vi "AWG Set and Arm.vi"(7 "pulse count (0: infinite)":i32, 8 "error in (no error)":errorcluster, 9 "trigger":T1, 10 "sampling rate":T5={"freq mode"=enum."fs or Ts", "fs [Hz]"=0.0, "fref [Hz]"=0.0, "mul"=0.0, "div"=0.0, "Amplitude (V)"=1.0}, 11 "awg session in":T7={"type"=enum."Agilent 331xxA to 332xxA", "VISA"="", "enable 10MHz ref"=FALSE, "cmi ckd2"={"VISA"="", "clock source"=enum."Auto", "manual ref clk"=FALSE, "ref clock [Hz]"=0.0, "div mode"=enum."Set divisor directly"}, "cmi sync v3"={"VISA"="", "baud rate [bd/s]"=115200, "source"=enum."Auto", "hv range"=enum."1kV", "fsrc is fixed"=FALSE, "fsrc [Hz]"=10000000.0, "freq integ [s]"=1.0, "freq filter"=5, "trig level"=enum."TTL 5V", "chn1 mode"=enum."Source divider", "chn1 level"=enum."Positive 5V", "chn2 mode"=enum."Source divider", "chn2 level"=enum."Positive 5V", "chn2 div"=1, "chn3 mode"=enum."Chn 1 Active", "chn3 level"=enum."Positive 5V", "chn1 div entry"=enum."Calculate nearest divisor from measured fx", "chn1 dev limit [%]"=1.0, "chn1 check dev"=FALSE}, "trigger"={"source"=enum."Immediate", "level [V]"=0.0, "coupling"=enum."DC", "slope"=enum."POS"}, "HMF2500 cfg"={"Baud Rate"=9600, "Parity"=0, "Data Bits"=8, "Flow Control"=4}} {"HMF2500 cfg"."Flow Control" items=["None", "XON/XOFF", "RTS/CTS", "XON/XOFF & RTS/CTS", "DTR/DSR", "XON/XOFF & DTR/DSR"]; "HMF2500 cfg"."Data Bits" items=["7"=7, "8"=8]; "HMF2500 cfg"."Parity" items=["None", "Odd", "Even", "Mark", "Space"]; "HMF2500 cfg"."Baud Rate" items=["300"=300, "600"=600, "1200"=1200, "2400"=2400, "4800"=4800, "9600"=9600, "19200"=19200]; "cmi sync v3"."chn2 div" min=1 max=100000000 step=1; "cmi sync v3"."fsrc [Hz]" format="%_8p"}) -> (0 "error out":errorcluster, 3 "awg session out":T7={"type"=enum."Agilent 331xxA to 332xxA", "VISA"="", "enable 10MHz ref"=FALSE, "cmi ckd2"={"VISA"="", "clock source"=enum."Auto", "manual ref clk"=FALSE, "ref clock [Hz]"=0.0, "div mode"=enum."Set divisor directly"}, "cmi sync v3"={"VISA"="", "baud rate [bd/s]"=115200, "source"=enum."Auto", "hv range"=enum."1kV", "fsrc is fixed"=FALSE, "fsrc [Hz]"=10000000.0, "freq integ [s]"=1.0, "freq filter"=5, "trig level"=enum."TTL 5V", "chn1 mode"=enum."Source divider", "chn1 level"=enum."Positive 5V", "chn2 mode"=enum."Source divider", "chn2 level"=enum."Positive 5V", "chn2 div"=1, "chn3 mode"=enum."Chn 1 Active", "chn3 level"=enum."Positive 5V", "chn1 div entry"=enum."Calculate nearest divisor from measured fx", "chn1 dev limit [%]"=1.0, "chn1 check dev"=FALSE}, "trigger"={"source"=enum."Immediate", "level [V]"=0.0, "coupling"=enum."DC", "slope"=enum."POS"}, "HMF2500 cfg"={"Baud Rate"=9600, "Parity"=0, "Data Bits"=8, "Flow Control"=4}} {"HMF2500 cfg"."Flow Control" items=["None", "XON/XOFF", "RTS/CTS", "XON/XOFF & RTS/CTS", "DTR/DSR", "XON/XOFF & DTR/DSR"]; "HMF2500 cfg"."Data Bits" items=["7"=7, "8"=8]; "HMF2500 cfg"."Parity" items=["None", "Odd", "Even", "Mark", "Space"]; "HMF2500 cfg"."Baud Rate" items=["300"=300, "600"=600, "1200"=1200, "2400"=2400, "4800"=4800, "9600"=9600, "19200"=19200]; "cmi sync v3"."chn2 div" min=1 max=100000000 step=1; "cmi sync v3"."fsrc [Hz]" format="%_8p"})   [LabVIEW 2020, in "AWG.lvlib"]
doc: "AWG wrapper: This sets the AWG to desired frequency and arms it. No pulses are generated here. Waiting for trigger!"
uses:
  AWG.lvlib
  AWG Session.ctl
  AWG Type.ctl
  CMI Clock Divider v2/CMI ckd2 Session.ctl
  CMI Clock Divider v2/CMI ckd2 Source Mode.ctl
  CMI Clock Divider v2/CMI ckd2 Divisor Mode.ctl
  CMI Sync V3/CMI Sync V3 session.ctl
  CMI Sync V3/Configure/CMI Sync V3 Reference Clock Source.ctl
  CMI Sync V3/Configure/CMI Sync V3 HV input Range.ctl
  CMI Sync V3/Configure/CMI Sync V3 Trigger Input Level.ctl
  CMI Sync V3/Configure/CMI Sync V3 Channel 1 Mode.ctl
  CMI Sync V3/Configure/CMI Sync V3 Channel Output Levels.ctl
  CMI Sync V3/Configure/CMI Sync V3 Channel 2 Mode.ctl
  CMI Sync V3/Configure/CMI Sync V3 Channel 3 Mode.ctl
  CMI Sync V3/Configure/CMI Sync V3 Channel 1 Divisor Entry Mode.ctl
  externals needed for AWG/ADC Trig Config.ctl
  externals needed for AWG/ADC Trig Mode Source.ctl
  externals needed for AWG/ADC Trig Coupling.ctl
  externals needed for AWG/ADC Trig Slope.ctl
  RaS HMF2500/HMF2500 Config.ctl
  externals needed for AWG/3458A Sampling Rate.ctl
  AWG Clock Setup Mode.ctl
  Agilent 33XXX Series/Agilent 33XXX Series.lvlib
  AFG3000/Tektronix AFG 3000 Series.lvlib
  CMI Sync V3/CMI Sync Unit V3.lvlib
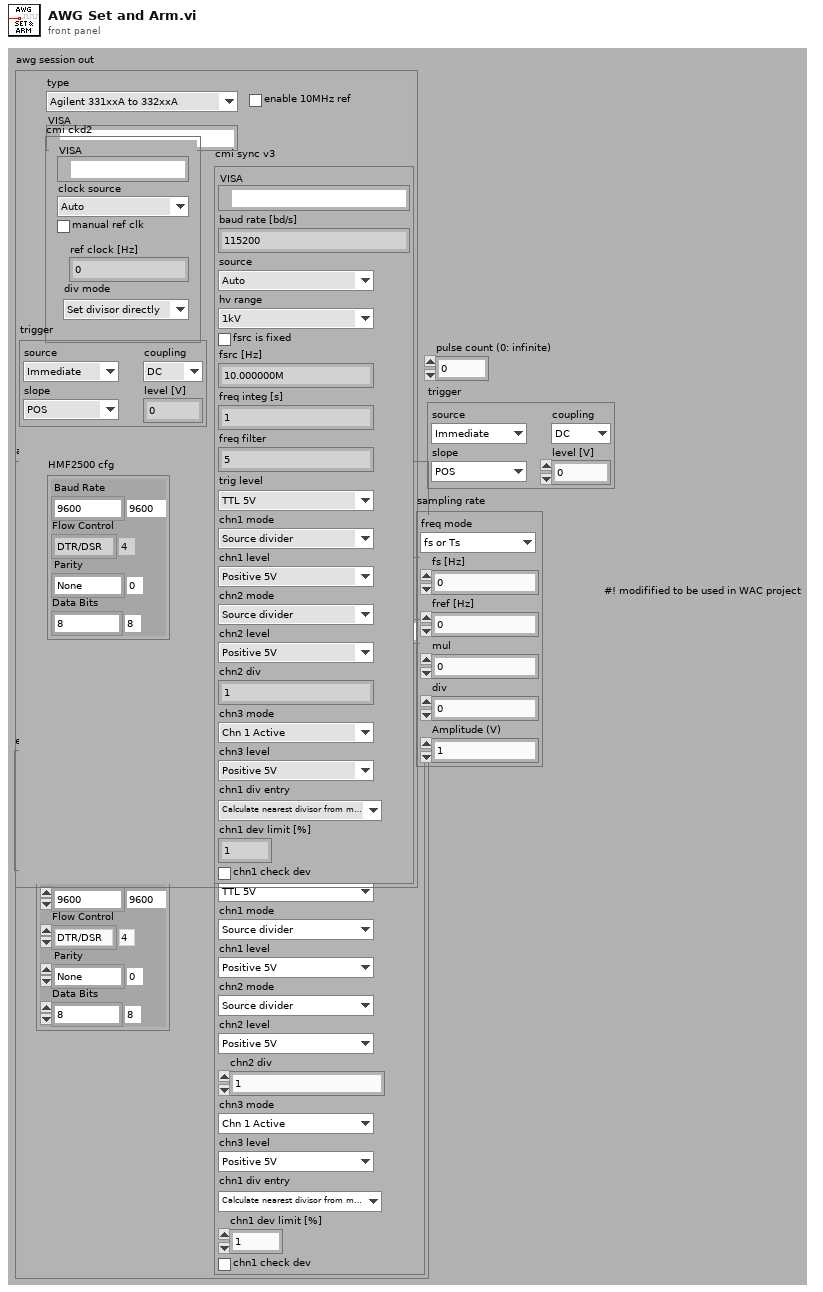
[diagram p1: front panel]
types:
  T1 = typedef "ADC Trig Config.ctl" = cluster{"source":T2, "level [V]":dbl, "coupling":T3, "slope":T4}
  T2 = typedef "ADC Trig Mode Source.ctl" = enum16{"Immediate", "External", "Level"}
  T3 = typedef "ADC Trig Coupling.ctl" = enum16{"DC", "AC"}
  T4 = typedef "ADC Trig Slope.ctl" = enum16{"POS", "NEG"}
  T5 = typedef "3458A Sampling Rate.ctl" = cluster{"freq mode":T6, "fs [Hz]":dbl, "fref [Hz]":dbl, "mul":dbl, "div":dbl, "Amplitude (V)":dbl}
  T6 = typedef "AWG.lvlib/AWG Clock Setup Mode.ctl" = enum16{"fs or Ts", "fs or Ts with fref", "fref/N", "fref*M/N", "fref*Ratio"}
  T7 = typedef "AWG.lvlib/AWG Session.ctl" = cluster{"type":T8, "VISA":refnum<visa-resource-name>, "enable 10MHz ref":bool, "cmi ckd2":T9, "cmi sync v3":T12, "trigger":T1, "HMF2500 cfg":T21}
  T8 = typedef "AWG.lvlib/AWG Type.ctl" = enum16{"Agilent 331xxA to 332xxA", "Agilent 335xxA to 336xxA", "Tektronix AFG3101C", "R&S HMF25xx", "CMI Clock Divider v2", "CMI Sync Unit V3", "dummy"}
  T9 = typedef "AWG.lvlib/CMI ckd2 Session.ctl" = cluster{"VISA":refnum<visa-resource-name>, "clock source":T10, "manual ref clk":bool, "ref clock [Hz]":dbl, "div mode":T11}
  T10 = typedef "AWG.lvlib/CMI ckd2 Source Mode.ctl" = enum16{"Auto", "LF clock", "HF clock", "Internal"}
  T11 = typedef "AWG.lvlib/CMI ckd2 Divisor Mode.ctl" = enum16{"Set divisor directly", "Set divisor by frequency"}
  T12 = typedef "AWG.lvlib/CMI Sync Unit V3.lvlib/CMI Sync V3 session.ctl" = cluster{"VISA":refnum<visa-resource-name>, "baud rate [bd/s]":i32, "source":T13, "hv range":T14, "fsrc is fixed":bool, "fsrc [Hz]":dbl, "freq integ [s]":dbl, "freq filter":i32, "trig level":T15, "chn1 mode":T16, "chn1 level":T17, "chn2 mode":T18, "chn2 level":T17, "chn2 div":i32, "chn3 mode":T19, "chn3 level":T17, "chn1 div entry":T20, "chn1 dev limit [%]":dbl, "chn1 check dev":bool}
  T13 = typedef "AWG.lvlib/CMI Sync Unit V3.lvlib/CMI Sync V3 Reference Clock Source.ctl" = enum16{"Auto", "Internal", "Logic", "Sine", "HV"}
  T14 = typedef "AWG.lvlib/CMI Sync Unit V3.lvlib/CMI Sync V3 HV input Range.ctl" = enum16{"10V", "60V", "250V", "1kV"}
  T15 = typedef "AWG.lvlib/CMI Sync Unit V3.lvlib/CMI Sync V3 Trigger Input Level.ctl" = enum16{"LVCMOS 3V3", "TTL 5V"}
  T16 = typedef "AWG.lvlib/CMI Sync Unit V3.lvlib/CMI Sync V3 Channel 1 Mode.ctl" = enum16{"Source divider", "DDS absolute", "DDS ratio", "DDS ratio M/N"}
  T17 = typedef "AWG.lvlib/CMI Sync Unit V3.lvlib/CMI Sync V3 Channel Output Levels.ctl" = enum16{"Positive 3V3", "Negative 3V3", "Positive 5V", "Negative 5V"}
  T18 = typedef "AWG.lvlib/CMI Sync Unit V3.lvlib/CMI Sync V3 Channel 2 Mode.ctl" = enum16{"Source divider", "Chn 1 divide"}
  T19 = typedef "AWG.lvlib/CMI Sync Unit V3.lvlib/CMI Sync V3 Channel 3 Mode.ctl" = enum16{"Chn 1 Active", "Chn 2 Active", "Chn 1 Trigger", "Chn 2 Trigger", "Gate", "PPS", "10MHz"}
  T20 = typedef "AWG.lvlib/CMI Sync Unit V3.lvlib/CMI Sync V3 Channel 1 Divisor Entry Mode.ctl" = enum16{"Set divisor directly", "Calculate nearest divisor from measured fx"}
  T21 = typedef "AWG.lvlib/HMF2500 Config.ctl" = cluster{"Baud Rate":u32, "Parity":u16, "Data Bits":u16, "Flow Control":u16}
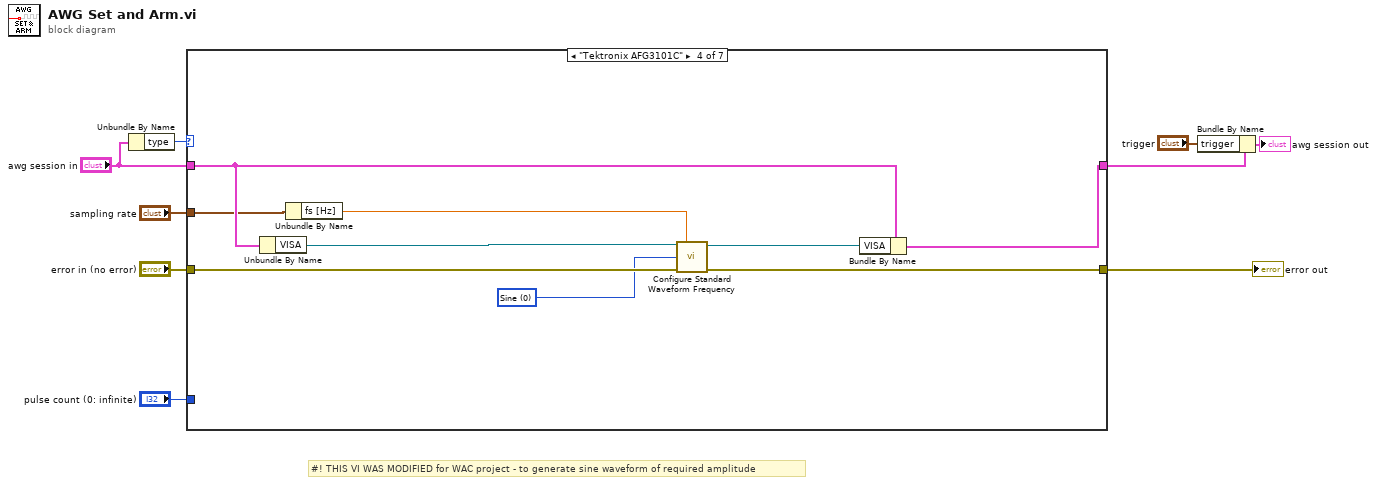
[diagram p0: block diagram]
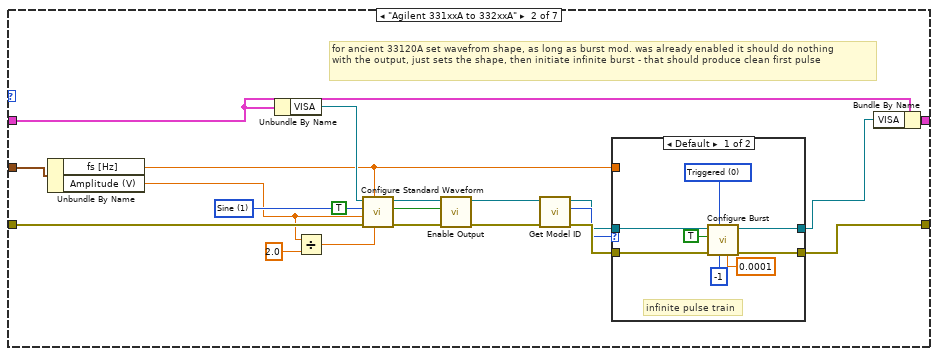
[diagram p3: hidden frame]
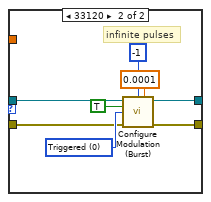
[diagram p4: hidden frame]
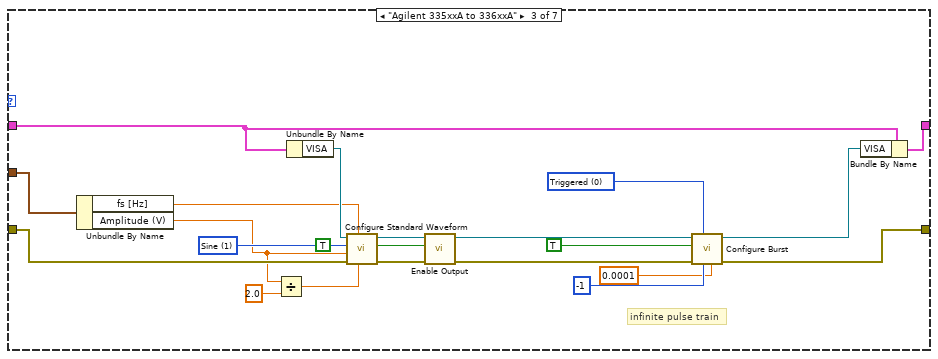
[diagram p5: hidden frame]
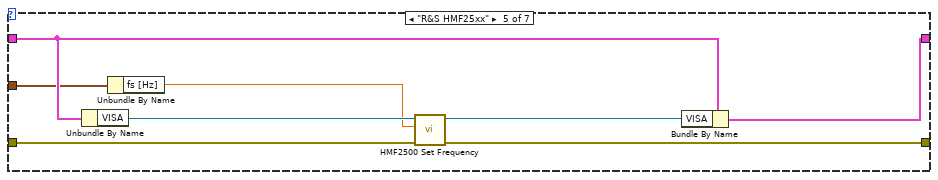
[diagram p6: hidden frame]
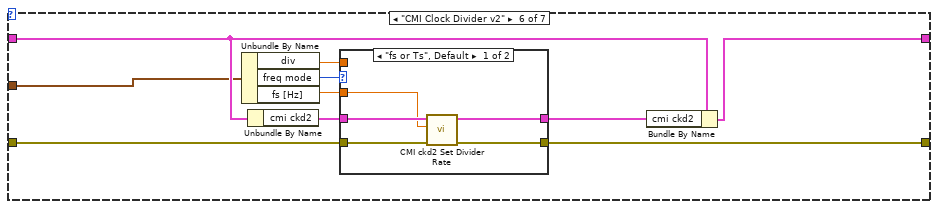
[diagram p7: hidden frame]
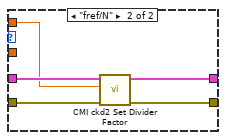
[diagram p8: hidden frame]
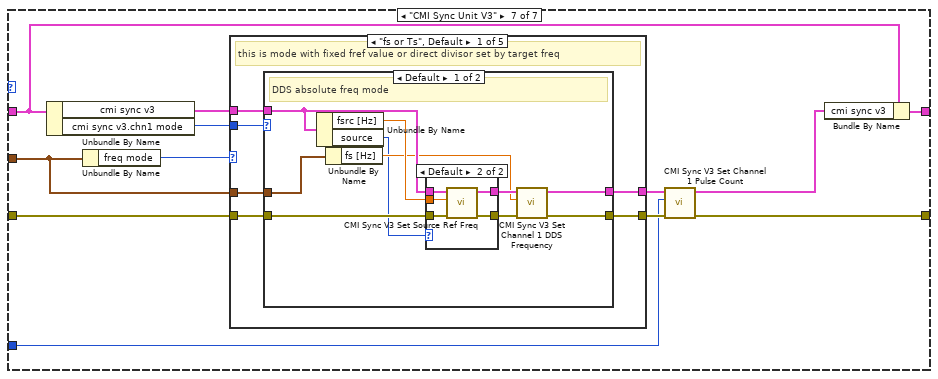
[diagram p9: hidden frame]
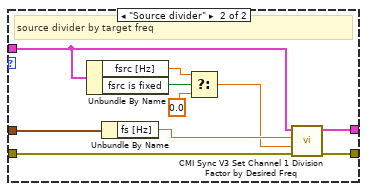
[diagram p11: hidden frame]
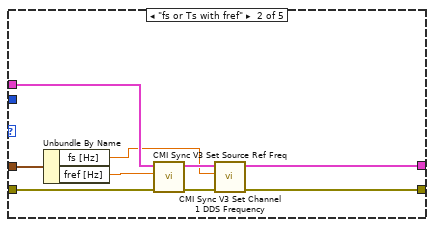
[diagram p12: hidden frame]
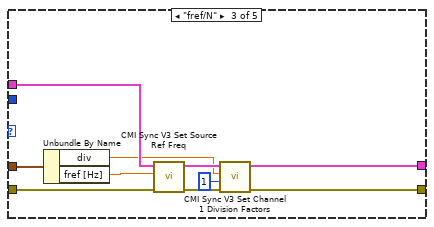
[diagram p13: hidden frame]
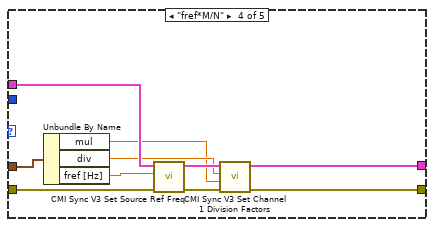
[diagram p14: hidden frame]
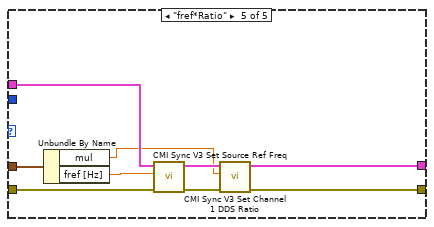
[diagram p15: hidden frame]
diagram:
  # "#! THIS VI WAS MODIFIED for WAC project - to generate sine waveform of required amplitude"
  n1 = Unbundle By Name("awg session in") -> ("type"=w9:T8)
  n2 = case shown="\"Tektronix AFG3101C\"" w9 {
    tunnel: "error in (no error)" -> [w11 w27 w60 w74 w82 w95 w116]
    tunnel: [w11 w17 w53 w71 w80 w90 w110] -> w7
    tunnel: "awg session in" -> [w10 w30 w68 w77 w85 w93 w112]
    tunnel: [w10 w31 w67 w76 w84 w89 w113] -> w4
    tunnel: "sampling rate" -> [_ w18 w61 w70 w79 w91 w114]
    tunnel: "pulse count (0: infinite)" -> [_ _ _ _ _ _ w109]
    frame Default {
    }
    frame "Agilent 331xxA to 332xxA" {
      w29 = u16 1 items=["DC", "Sine", "Square", "Triangle", "Ramp", "Pulse", "Noise", "Sinc", "Negative Ramp", "Exponential Rise", "Exponential Fall", "Cardiac"] ("Waveform Function (1: Sine)")
      # "for ancient 33120A set wavefrom shape, as long as burst mod. was already enabled it should do nothing\nwith the output, just sets the shape, then initiate infinite burst - that should produce clean first pulse"
      n3 = Unbundle By Name(w18) -> ("fs [Hz]"=w15:dbl, "Amplitude (V)"=w13:dbl)
      n4 = Unbundle By Name(w30) -> ("VISA"=w28:refnum<visa-resource-name>)
      n5 = Divide(x=w13, y=2.0 ("DC Offset (0.00 V)")) -> (x/y=w12:dbl)
      n6 = call "Configure Standard Waveform.vi"("DC Offset (0.00 V)"=w12, "Frequency (1000 Hz)"=w15, "error in (no error)"=w27, "Amplitude (1)"=w13, "Waveform Function (1: Sine)"=w29, "VISA resource name"=w28) -> ("error out"=w26:errorcluster, "VISA resource name out"=w25:refnum<visa-resource-name>)  [unwired: 4 in]
      n7 = call "Enable Output.vi"("error in (no error)"=w26, "Enable Output  (T: Enable)"=TRUE, "VISA resource name"=w25) -> ("error out"=w23:errorcluster, "VISA resource name out"=w22:refnum<visa-resource-name>)  [unwired: 7 in]
      n8 = call "Get Model ID.vi"("error in (no error)"=w23, "VISA resource name"=w22) -> ("error out"=w21:errorcluster, "model ID"=w20:u32, "VISA resource name out"=w19:refnum<visa-resource-name>)  [unwired: 7 in]
      n9 = case shown="Default" w20 {
        tunnel: [w38 w44] -> w17
        tunnel: [w37 w43] -> w16
        tunnel: w15 -> [_ _]
        tunnel: w21 -> [w39 w42]
        tunnel: w19 -> [w36 w41]
        frame Default {
          w35 = u16 0 items=["Triggered", "Gated"] ("Burst Mode (0: Triggered)")
          # "infinite pulse train"
          n10 = call "Configure Burst.vi"("Burst Period (1 s)"=0.0001, "Burst Count (1)"=-1, "Burst Mode (0: Triggered)"=w35, "error in (no error)"=w39, "Enable Burst (T: Enable)"=TRUE, "VISA resource name"=w36) -> ("error out"=w38:errorcluster, "VISA resource name out"=w37:refnum<visa-resource-name>)  [unwired: 4 in]
        }
        frame 33120 {
          w45 = u16 0 items=["Triggered", "Gated"] ("Burst Modulation Mode (0: Triggered)")
          # "infinite pulses"
          n11 = call "Configure Modulation (Burst).vi"("VISA resource name"=w41, "Burst Count (1)"=-1, "Burst Period (1 s)"=0.0001, "Enable Burst Modulation (T: Enable)"=TRUE, "Burst Modulation Mode (0: Triggered)"=w45, "error in (no error)"=w42) -> ("VISA resource name out"=w43:refnum<visa-resource-name>, "error out"=w44:errorcluster)  [unwired: 8 in]
        }
      }
      n12 = Bundle By Name(cluster=w30, "VISA"=w16) -> (w31:T7)
    }
    frame "Agilent 335xxA to 336xxA" {
      w59 = u16 0 items=["Triggered", "Gated"] ("Burst Mode (0: Triggered)")
      w66 = u16 1 items=["DC", "Sine", "Square", "Triangle", "Ramp", "Pulse", "Noise", "Sinc", "Negative Ramp", "Exponential Rise", "Exponential Fall", "Cardiac"] ("Waveform Function (1: Sine)")
      # "infinite pulse train"
      n13 = Unbundle By Name(w61) -> ("fs [Hz]"=w51:dbl, "Amplitude (V)"=w49:dbl)
      n14 = Divide(x=w49, y=2.0 ("DC Offset (0.00 V)")) -> (x/y=w48:dbl)
      n15 = Unbundle By Name(w68) -> ("VISA"=w62:refnum<visa-resource-name>)
      n16 = call "Configure Standard Waveform.vi"("DC Offset (0.00 V)"=w48, "Frequency (1000 Hz)"=w51, "error in (no error)"=w60, "Amplitude (1)"=w49, "Waveform Function (1: Sine)"=w66, "VISA resource name"=w62) -> ("error out"=w65:errorcluster, "VISA resource name out"=w64:refnum<visa-resource-name>)  [unwired: 4 in]
      n17 = call "Enable Output.vi"("error in (no error)"=w65, "Enable Output  (T: Enable)"=TRUE, "VISA resource name"=w64) -> ("error out"=w55:errorcluster, "VISA resource name out"=w54:refnum<visa-resource-name>)  [unwired: 7 in]
      n18 = call "Configure Burst.vi"("Burst Period (1 s)"=0.0001, "Burst Count (1)"=-1, "Burst Mode (0: Triggered)"=w59, "error in (no error)"=w55, "Enable Burst (T: Enable)"=TRUE, "VISA resource name"=w54) -> ("error out"=w53:errorcluster, "VISA resource name out"=w52:refnum<visa-resource-name>)  [unwired: 4 in]
      n19 = Bundle By Name(cluster=w68, "VISA"=w52) -> (w67:T7)
    }
    frame "Tektronix AFG3101C" {
      w73 = u16 0 items=["Sine", "Square", "Pulse", "Ramp", "Noise", "DC", "Sin(x)/x", "Gaussian", "Lorentz", "Exponential Rise", "Exponential Decay", "Haversine"] ("Waveform Function (0: Sine)")
      n20 = Unbundle By Name(w77) -> ("VISA"=w75:refnum<visa-resource-name>)
      n21 = Unbundle By Name(w70) -> ("fs [Hz]"=w69:dbl)
      n22 = call "Configure Standard Waveform Frequency.vi"("VISA resource name"=w75, "Frequency (1000 Hz)"=w69, "Waveform Function (0: Sine)"=w73, "error in (no error)"=w74) -> ("VISA resource name out"=w72:refnum<visa-resource-name>, "error out"=w71:errorcluster)  [unwired: 10 in]
      n23 = Bundle By Name(cluster=w77, "VISA"=w72) -> (w76:T7)
    }
    frame "R&S HMF25xx" {
      n24 = Unbundle By Name(w85) -> ("VISA"=w83:refnum<visa-resource-name>)
      n25 = Unbundle By Name(w79) -> ("fs [Hz]"=w78:dbl)
      n26 = call "HMF2500 Set Frequency.vi"("error in (no error)"=w82, "frequency [Hz] (1000)"=w78, "VISA in"=w83) -> ("error out"=w80:errorcluster, "VISA out"=w81:refnum<visa-resource-name>)  [unwired: 7 in]
      n27 = Bundle By Name(cluster=w85, "VISA"=w81) -> (w84:T7)
    }
    frame "CMI Clock Divider v2" {
      n28 = Unbundle By Name(w91) -> ("div"=w86:dbl, "freq mode"=w87:T6, "fs [Hz]"=w88:dbl)
      n29 = Unbundle By Name(w93) -> ("cmi ckd2"=w94:T9)
      n30 = case shown="\"fs or Ts\", Default" w87 {
        tunnel: w95 -> [w100 w105]
        tunnel: w94 -> [w98 w102]
        tunnel: [w96 w103] -> w92
        tunnel: [w99 w104] -> w90
        tunnel: w88 -> [w97 _]
        tunnel: w86 -> [_ w101]
        frame "fs or Ts", Default {
          n31 = call "CMI ckd2 Set Divider Rate.vi"("error in"=w100, "clock rate [Hz]"=w97, "session"=w98) -> ("error out"=w99:errorcluster, "session out"=w96:T9)  [unwired: 5 in, 2 out]
        }
        frame "fref/N" {
          n32 = call "CMI ckd2 Set Divider Factor.vi"("error in"=w105, "division factor (1)"=w101, "session"=w102) -> ("error out"=w104:errorcluster, "session out"=w103:T9)  [unwired: 7 in]
        }
      }
      n33 = Bundle By Name(cluster=w93, "cmi ckd2"=w92) -> (w89:T7)
    }
    frame "CMI Sync Unit V3" {
      n34 = Unbundle By Name(w112) -> ("cmi sync v3"=w115:T12, "cmi sync v3.chn1 mode"=w106:T16)
      n35 = Unbundle By Name(w114) -> ("freq mode"=w117:T6)
      n36 = case shown="\"fs or Ts\", Default" w117 {
        tunnel: w116 -> [w123 w159 w169 w179 w188]
        tunnel: w115 -> [w119 w158 w168 w178 w187]
        tunnel: w114 -> [w122 w156 w166 w176 w185]
        tunnel: [w121 w153 w163 w173 w182] -> w111
        tunnel: [w120 w152 w162 w172 w181] -> w108
        tunnel: w106 -> [w118 _ _ _ _]
        frame "fs or Ts", Default {
          # "this is mode with fixed fref value or direct divisor set by target freq"
          n37 = case shown="Default" w118 {
            tunnel: w123 -> [w133 w150]
            tunnel: w122 -> [w131 w149]
            tunnel: [w129 w147] -> w121
            tunnel: [w128 w146] -> w120
            tunnel: w119 -> [w127 w145]
            frame Default {
              # "DDS absolute freq mode"
              n38 = Unbundle By Name(w127) -> ("fsrc [Hz]"=w126:dbl, "source"=w124:T13)
              n39 = Unbundle By Name(w131) -> ("fs [Hz]"=w125:dbl)
              n40 = case shown="Default" w124 {
                tunnel: w133 -> [w135 w140]
                tunnel: [w135 w139] -> w132
                tunnel: [w134 w138] -> w130
                tunnel: w127 -> [w134 w137]
                tunnel: w126 -> [_ w136]
                frame "Internal" {
                }
                frame Default {
                  n41 = call "CMI Sync V3 Set Source Ref Freq.vi"("error in"=w140, "Expected reference frequency [Hz]"=w136, "session in"=w137) -> ("error out"=w139:errorcluster, "session out"=w138:T12)  [unwired: 7 in]
                }
              }
              n42 = call "CMI Sync V3 Set Channel 1 DDS Frequency.vi"("error in"=w132, "DDS absolute [Hz] (1 MHz)"=w125, "session in"=w130) -> ("error out"=w129:errorcluster, "session out"=w128:T12)  [unwired: 7 in]
            }
            frame "Source divider" {
              # "source divider by target freq"
              n43 = Unbundle By Name(w145) -> ("fsrc [Hz]"=w143:dbl, "fsrc is fixed"=w144:bool)
              n44 = Unbundle By Name(w149) -> ("fs [Hz]"=w148:dbl)
              n45 = Select(t=w143, s=w144, f=0.0) -> (s? t:f=w141:dbl)
              n46 = call "CMI Sync V3 Set Channel 1 Division Factor by Desired Freq.vi"("error in"=w150, "explicit ref freq [Hz] (0: auto estimate)"=w141, "target output freq [Hz]"=w148, "session in"=w145) -> ("error out"=w147:errorcluster, "session out"=w146:T12)  [unwired: 4 in, 2 out]
            }
          }
        }
        frame "fs or Ts with fref" {
          n47 = Unbundle By Name(w156) -> ("fs [Hz]"=w151:dbl, "fref [Hz]"=w155:dbl)
          n48 = call "CMI Sync V3 Set Source Ref Freq.vi"("error in"=w159, "Expected reference frequency [Hz]"=w155, "session in"=w158) -> ("error out"=w157:errorcluster, "session out"=w154:T12)  [unwired: 7 in]
          n49 = call "CMI Sync V3 Set Channel 1 DDS Frequency.vi"("error in"=w157, "DDS absolute [Hz] (1 MHz)"=w151, "session in"=w154) -> ("error out"=w153:errorcluster, "session out"=w152:T12)  [unwired: 7 in]
        }
        frame "fref/N" {
          n50 = Unbundle By Name(w166) -> ("div"=w161:dbl, "fref [Hz]"=w165:dbl)
          n51 = call "CMI Sync V3 Set Source Ref Freq.vi"("error in"=w169, "Expected reference frequency [Hz]"=w165, "session in"=w168) -> ("error out"=w167:errorcluster, "session out"=w164:T12)  [unwired: 7 in]
          n52 = call "CMI Sync V3 Set Channel 1 Division Factors.vi"("error in"=w167, "DDS multiplier (1)"=1, "Divider (10)"=w161, "session in"=w164) -> ("error out"=w163:errorcluster, "session out"=w162:T12)  [unwired: 6 in]
        }
        frame "fref*M/N" {
          n53 = Unbundle By Name(w176) -> ("mul"=w170:dbl, "div"=w171:dbl, "fref [Hz]"=w175:dbl)
          n54 = call "CMI Sync V3 Set Source Ref Freq.vi"("error in"=w179, "Expected reference frequency [Hz]"=w175, "session in"=w178) -> ("error out"=w177:errorcluster, "session out"=w174:T12)  [unwired: 7 in]
          n55 = call "CMI Sync V3 Set Channel 1 Division Factors.vi"("error in"=w177, "DDS multiplier (1)"=w170, "Divider (10)"=w171, "session in"=w174) -> ("error out"=w173:errorcluster, "session out"=w172:T12)  [unwired: 6 in]
        }
        frame "fref*Ratio" {
          n56 = Unbundle By Name(w185) -> ("mul"=w180:dbl, "fref [Hz]"=w184:dbl)
          n57 = call "CMI Sync V3 Set Source Ref Freq.vi"("error in"=w188, "Expected reference frequency [Hz]"=w184, "session in"=w187) -> ("error out"=w186:errorcluster, "session out"=w183:T12)  [unwired: 7 in]
          n58 = call "CMI Sync V3 Set Channel 1 DDS Ratio.vi"("error in"=w186, "DDS ratio (1.0)"=w180, "session in"=w183) -> ("error out"=w182:errorcluster, "session out"=w181:T12)  [unwired: 7 in]
        }
      }
      n59 = call "CMI Sync V3 Set Channel 1 Pulse Count.vi"("error in"=w111, "Pulse count (0: infinite)"=w109, "session in"=w108) -> ("error out"=w110:errorcluster, "session out"=w107:T12)  [unwired: 7 in]
      n60 = Bundle By Name(cluster=w112, "cmi sync v3"=w107) -> (w113:T7)
    }
  }
  "error out" <- w7
  n61 = Bundle By Name(cluster=w4, "trigger"="trigger") -> (→"awg session out":T7)
